vi "close accessory panels.vi"(8 "error in (no error)":errorcluster, 11 "refs":T1) -> (0 "error out":errorcluster)   [LabVIEW 2010]
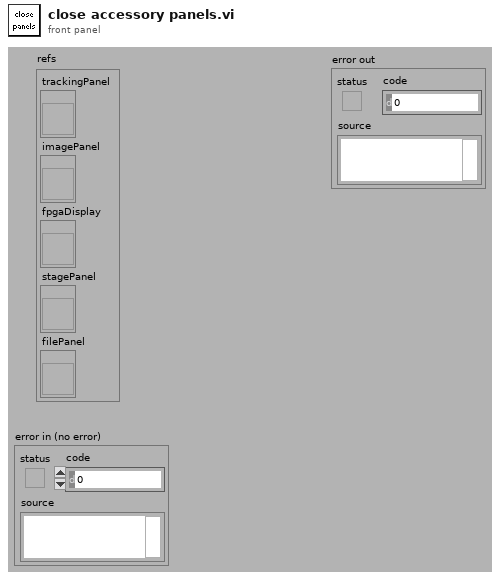
[diagram p1: front panel]
types:
  T1 = cluster{"trackingPanel":refnum<vi>, "imagePanel":refnum<vi>, "fpgaDisplay":refnum<vi>, "stagePanel":refnum<vi>, "filePanel":refnum<vi>}
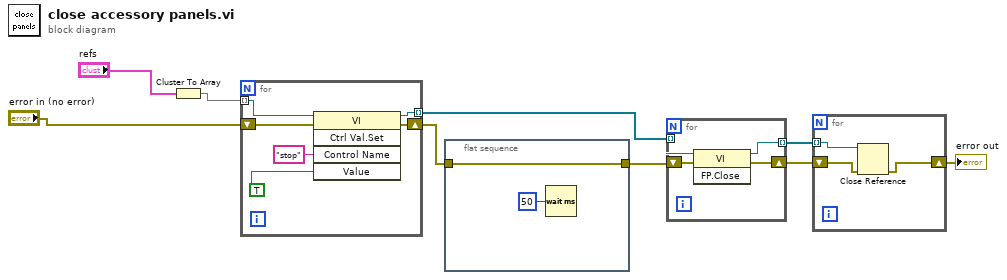
[diagram p0: block diagram]
diagram:
  n1 = Cluster To Array(cluster="refs") -> (array=w7:refnum<vi>[])
  n2 = for {
    tunnel: w7 -> [w12] mode=indexing
    shift-right: [w11] -> w6
    shift-left: "error in (no error)" -> [w15]
    tunnel: [w10] -> w4 mode=indexing
    n3 = invoke class="VI" method="Ctrl Val.Set"(reference=w12, error in=w15, "Control Name"="stop", "Value"=TRUE ("stop")) -> (reference out=w10:refnum<vi>, error out=w11:errorcluster)  [unwired: 1 in, 3 out]
  }
  n4 = flat-sequence {
    tunnel: w6 -> [w16]
    tunnel: [w16] -> w5
    frame #0 {
      n5 = Wait (ms)(milliseconds to wait=u32 50) -> ()  [unwired: 1 out]
    }
  }
  n6 = for {
    tunnel: w4 -> [w20] mode=indexing
    shift-right: [w19] -> w3
    shift-left: w5 -> [w21]
    tunnel: [w18] -> w2 mode=indexing
    n7 = invoke class="VI" method="FP.Close"(reference=w20, error in=w21) -> (reference out=w18:refnum<vi>, error out=w19:errorcluster)  [unwired: 1 in, 1 out]
  }
  n8 = for {
    shift-right: [w22] -> w1
    shift-left: w3 -> [w24]
    tunnel: w2 -> [w23] mode=indexing
    n9 = Close Reference(reference=w23, error in (no error)=w24) -> (error out=w22:errorcluster)
  }
  "error out" <- w1
